vi "TEMOCR-Compute Gain.vi"(0 "State In":T1, 5 "Analysis":T2, 9 "seqIndex":i32) -> (4 "State Out":T1, 8 "freq response":cluster{"Freq (Hz)":dbl[], "Mag (dB)":dbl[]})   [LabVIEW 2015]
uses:
  Typedefs/TEMOCR-Analysis.ctl
  Typedefs/TEMOCR-Analysis State.ctl
  <vilib>/Analysis/baseanly.llb/Mean (DBL).vi
  Utility VIs/Array Manipulation VIs/Irregular Array Subset (DBL).vi
  Utility VIs/Math VIs/dB to Linear (1D).vi
  Utility VIs/Math VIs/Linear to dB (scalar).vi
  <vilib>/Analysis/NI_AALBase.lvlib
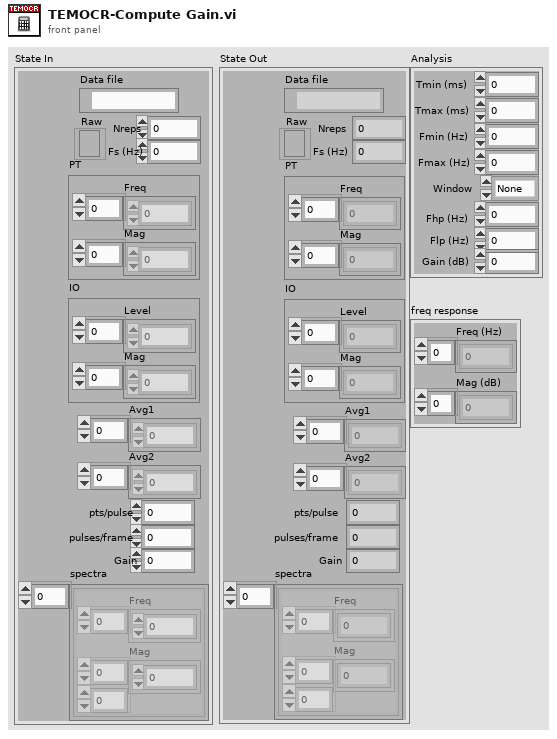
[diagram p1: front panel]
types:
  T1 = typedef "TEMOCR-Analysis State.ctl" = cluster{"Data file":path, "Raw":refnum<file>, "PT":cluster{"Freq":dbl[], "Mag":dbl[]}, "IO":cluster{"Level":dbl[], "Mag":dbl[]}, "Nreps":i32, "Fs (Hz)":dbl, "Avg1":dbl[], "pts/pulse":i32, "pulses/frame":i32, "Avg2":dbl[], "Gain":dbl, "spectra":cluster{"Freq":dbl[], "Mag":dbl[][]}[]}
  T2 = typedef "TEMOCR-Analysis.ctl" = cluster{"Tmin (ms)":dbl, "Tmax (ms)":dbl, "Fmin (Hz)":dbl, "Fmax (Hz)":dbl, "Window":enum16{"None", "Hanning", "Hamming"}, "Fhp (Hz)":dbl, "Flp (Hz)":dbl, "Gain (dB)":dbl}
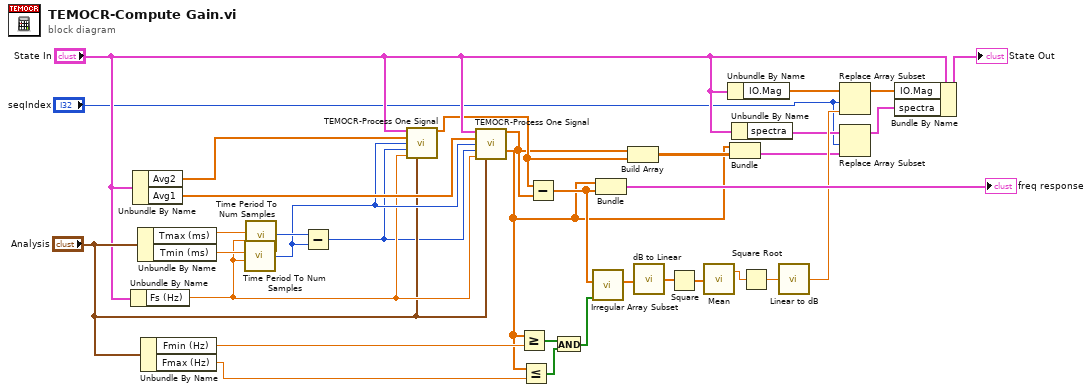
[diagram p0: block diagram]
diagram:
  n1 = Unbundle By Name("State In") -> ("Fs (Hz)"=w13:dbl)
  n2 = Unbundle By Name("State In") -> ("Avg2"=w16:dbl[], "Avg1"=w15:dbl[])
  n3 = Unbundle By Name("Analysis") -> ("Tmax (ms)"=w18:dbl, "Tmin (ms)"=w19:dbl)
  n4 = Unbundle By Name("Analysis") -> ("Fmin (Hz)"=w33:dbl, "Fmax (Hz)"=w32:dbl)
  n5 = call "Time Period To Num Samples.vi"("Duration (ms)"=w19, "Sampling rate (Hz)"=w13) -> ("Samples"=w14:i32)  [unwired: 5 in]
  n6 = call "Time Period To Num Samples.vi"("Duration (ms)"=w18, "Sampling rate (Hz)"=w13) -> ("Samples"=w17:i32)  [unwired: 5 in]
  n7 = Subtract(x=w17, y=w14) -> (x-y=w1:i32)
  n8 = call "TEMOCR-Process One Signal.vi"("State In"="State In", "array"=w16, "index"=w14, "length"=w1, "Fs (Hz)"=w13, "Analysis"="Analysis") -> ("+Freq. Mag of FFT (dB rms)"=w9:dbl[])  [unwired: 8 in, 1 out]
  n9 = call "TEMOCR-Process One Signal.vi"("State In"="State In", "array"=w15, "index"=w14, "length"=w1, "Fs (Hz)"=w13, "Analysis"="Analysis") -> ("+Freq. Mag of FFT (dB rms)"=w7:dbl[], "Freq (Hz)"=w6:dbl[])  [unwired: 8 in]
  n10 = Greater Or Equal?(x=w6, y=w33) -> (x >= y?=w31:bool[])
  n11 = Less Or Equal?(x=w6, y=w32) -> (x <= y?=w30:bool[])
  n12 = Subtract(x=w9, y=w7) -> (x-y=w11:dbl[])
  n13 = And(x=w31, y=w30) -> (x .and. y?=w29:bool[])
  n14 = call-poly "Irregular Array Subset.vi"("Mask"=w29, "Array"=w11) -> ("Array Subset"=w28:dbl[])  [unwired: 8 in, 1 out]
  n15 = Bundle("Freq (Hz)"=w6, w11) -> (→"freq response":cluster{"Freq (Hz)":dbl[], dbl[]})  [unwired: 1 in]
  n16 = Build Array(w7, w9) -> (w8:dbl[][])
  n17 = call-poly "dB to Linear.vi"("dB"=w28) -> ("linear"=w27:dbl[])
  n18 = Square(x=w27) -> (x^2=w26:dbl[])
  n19 = call-poly <vilib>:"Mean.vi"("X"=w26) -> ("mean"=w25:dbl)  [unwired: 1 out]
  n20 = Unbundle By Name("State In") -> ("IO.Mag"=w23:dbl[])
  n21 = Bundle("Freq (Hz)"=w6, w8) -> (w3:cluster{"Freq (Hz)":dbl[], dbl[][]})  [unwired: 1 in]
  n22 = Unbundle By Name("State In") -> ("spectra"=w5:cluster{"Freq":dbl[], "Mag":dbl[][]}[])
  n23 = Square Root(x=w25) -> (sqrt(x)=w24:dbl)
  n24 = call-poly "Linear to dB.vi"("Linear"=w24) -> ("dB"=w22:dbl)
  n25 = Replace Array Subset(array=w23, new element=w22, index="seqIndex") -> (w20:dbl[])
  n26 = Replace Array Subset(array=w5, new element=w3, index="seqIndex") -> (w2:cluster{"Freq":dbl[], "Mag":dbl[][]}[])
  n27 = Bundle By Name(cluster="State In", "IO.Mag"=w20, "spectra"=w2) -> (→"State Out":T1)
